vi "Fill_Measur_Buffer.vi"(4 "[IN] Current Measure":dbl, 5 "[IN] Current Index":i32, 7 "[IN] Buffer":dbl[](array[numeric])) -> (1 "[OUT] Current Index":i32, 3 "[OUT] Buffer":dbl[](array[numeric]))   [LabVIEW 2022 SP3]
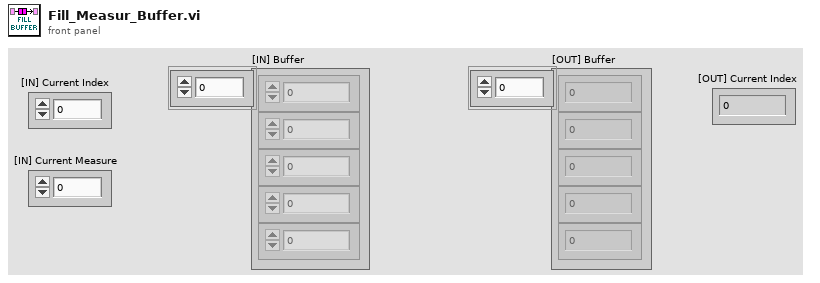
[diagram p1: front panel]
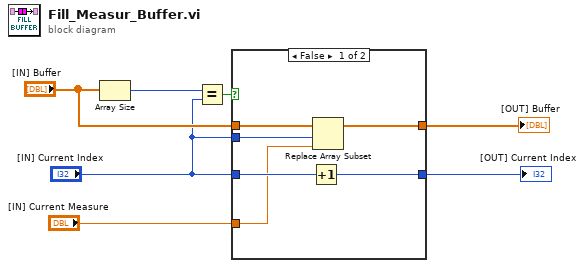
[diagram p0: block diagram]
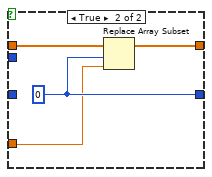
[diagram p2: hidden frame]
diagram:
  n1 = Array Size(array="[IN] Buffer") -> (size(s)=w1:i32)
  n2 = Equal?(x=w1, y="[IN] Current Index") -> (x = y?=w7:bool)
  n3 = case shown="False" w7 {
    tunnel: "[IN] Buffer" -> [w11 w17]
    tunnel: "[IN] Current Index" -> [w9 _]
    tunnel: "[IN] Current Measure" -> [w8 w14]
    tunnel: [w10 w16] -> w4
    tunnel: "[IN] Current Index" -> [w13 _]
    tunnel: [w12 w15] -> w2
    frame False {
      n4 = Increment(x=w13) -> (x+1=w12:i32)
      n5 = Replace Array Subset(array=w11, new element=w8, index=w9) -> (w10:dbl[])
    }
    frame True {
      w15 = 0
      n6 = Replace Array Subset(array=w17, new element=w14, index=w15) -> (w16:dbl[])
    }
  }
  "[OUT] Buffer" <- w4
  "[OUT] Current Index" <- w2
